vi "Autonomous Shooting.vi"(6 "Cross Obstacle":bool, 7 "Ball in place":bool, 8 "The Desired":T1={"Desired Angle"=45.0, "Desired Distance"=30.0, "Desired Time"=4.0}, 9 "Sensor Values":T2, 10 "Goal Selection":cluster{"High Goal":bool, "Low Goal":bool}, 11 "Position Selection":T6) -> (0 "Complete":bool, 1 "Arcada Drive?":bool, 2 "Tank Drive":T4, 3 "Aracade Drive":T5)   [LabVIEW 2015]
uses:
  Autonomous Shooting States.ctl
  Sensors.vi
panel:
  in  "Desired Angle for Position 2":dbl
  in  "Speed":dbl=0.4
  out "Set Roller/Shoot Motor":T3
  in  "X axis value":dbl=0.3
  # "12.27272727272727271"
  # "12.27272727272727271"
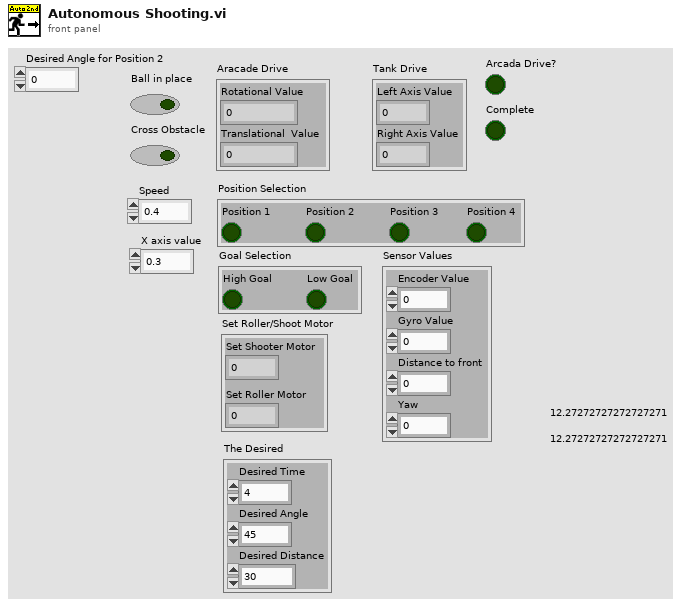
[diagram p1: front panel]
types:
  T1 = cluster{"Desired Angle":dbl, "Desired Distance":dbl, "Desired Time":dbl}
  T2 = cluster{"Encoder Value":dbl, "Gyro Value":dbl, "Distance to front":dbl, "Yaw":dbl}
  T3 = cluster{"Set Shooter Motor":dbl, "Set Roller Motor":dbl}
  T4 = cluster{"Left Axis Value":dbl, "Right Axis Value":dbl}
  T5 = cluster{"Rotational Value":dbl, "Translational  Value":dbl}
  T6 = cluster{"Position 1":bool, "Position 2":bool, "Position 3":bool, "Position 4":bool}
  T7 = typedef "Autonomous Shooting States.ctl" = enum16{"Ready", "Correct Heading", "Zero Encoder", "Drive Forward for X", "Turn towards goal 1", "Turn towards goal 2", "Turn towards goal 3", "Drive to Castle", "Check goal", "High Goal", "Positioning", "Low Goal", "Complete"}
  T8 = cluster{"Rotational Value":dbl, "Rotational Value":dbl}
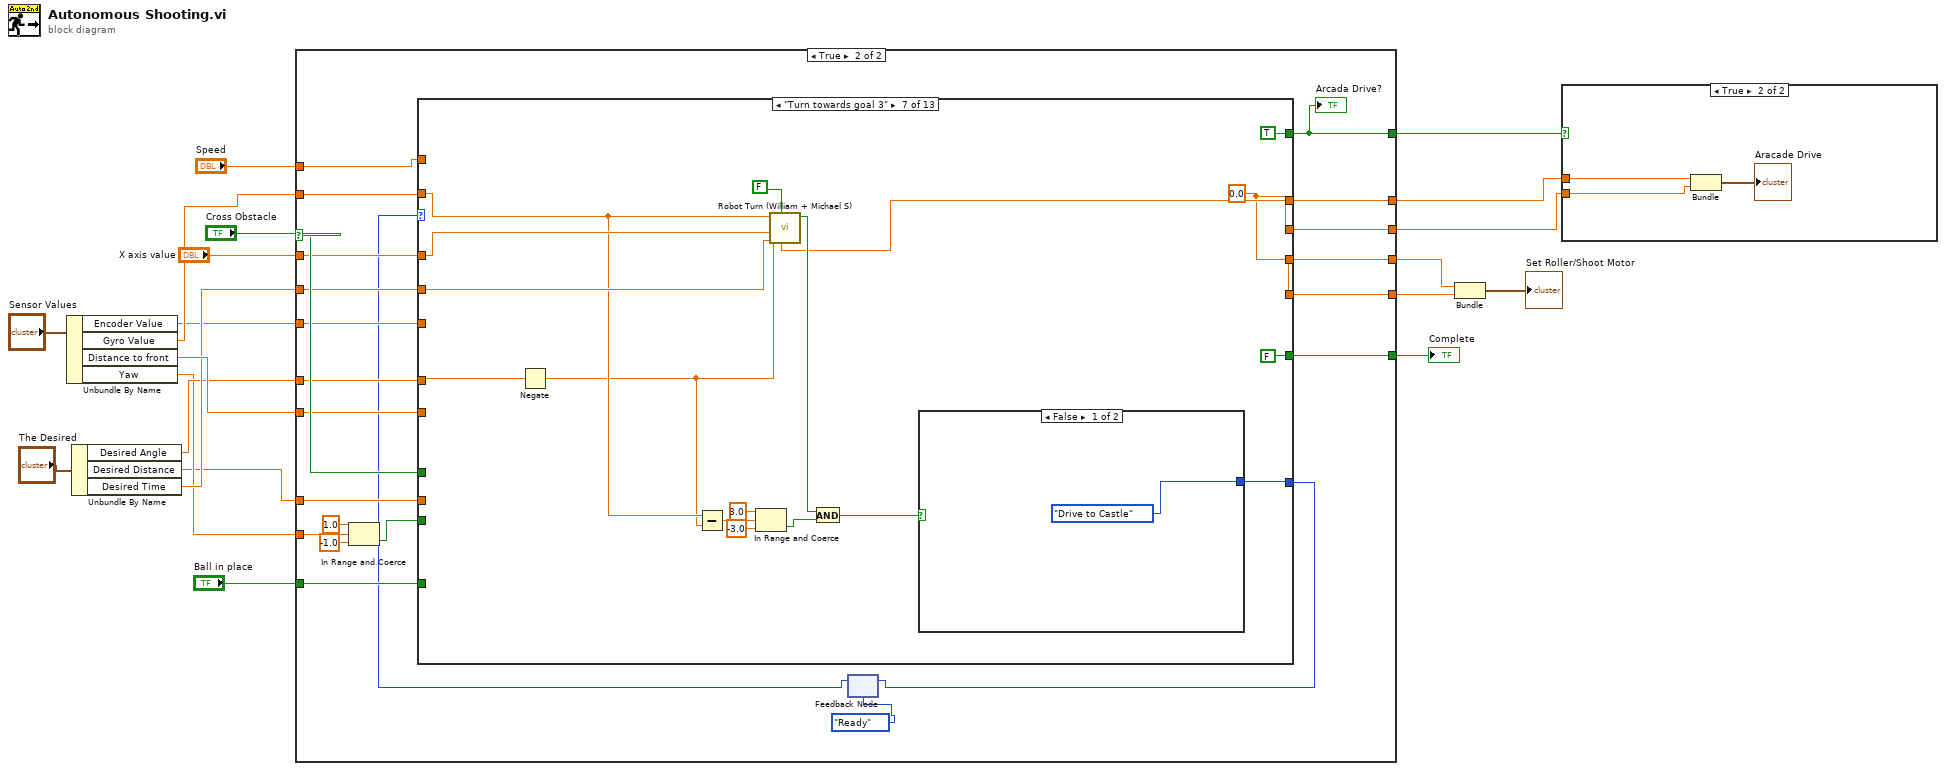
[diagram p0: block diagram]
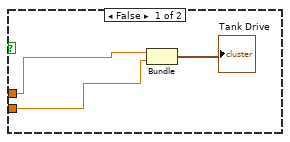
[diagram p2: hidden frame]
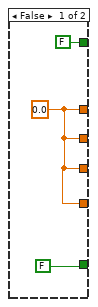
[diagram p3: hidden frame]
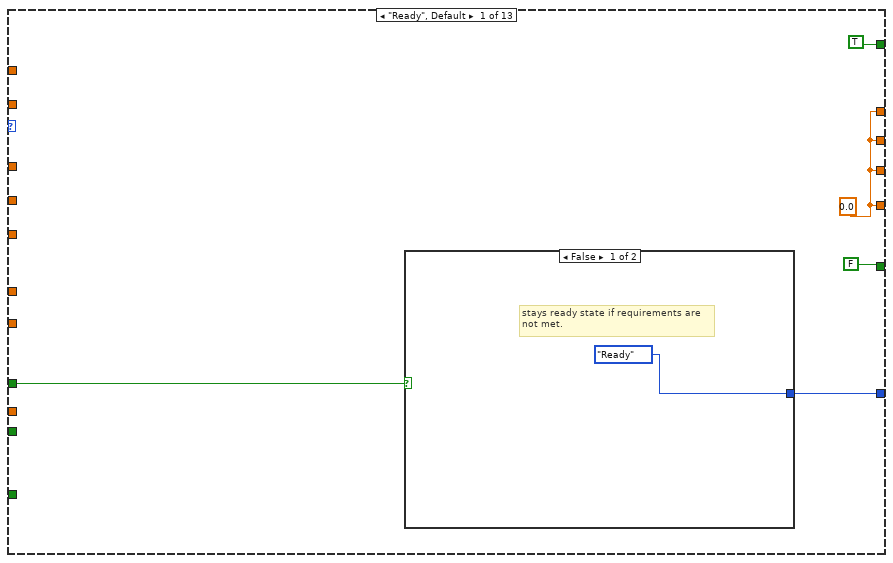
[diagram p4: hidden frame]
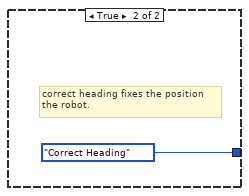
[diagram p5: hidden frame]
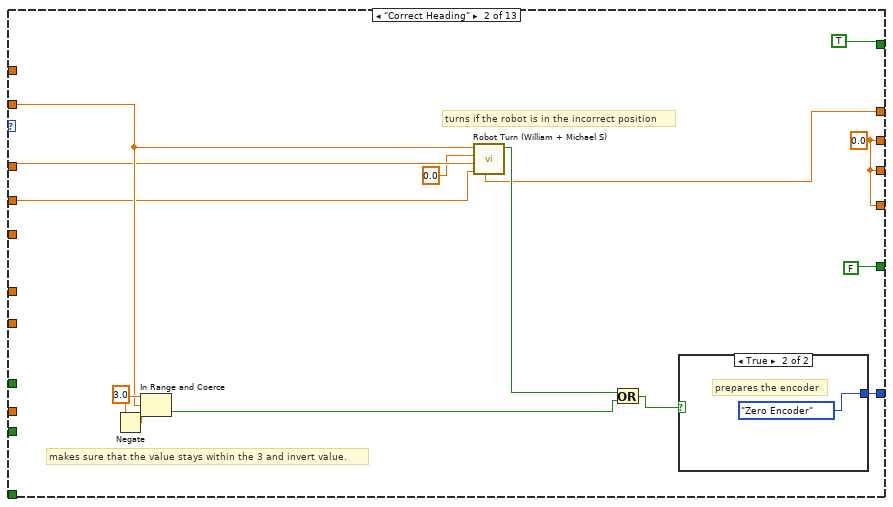
[diagram p6: hidden frame]
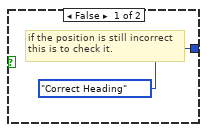
[diagram p7: hidden frame]
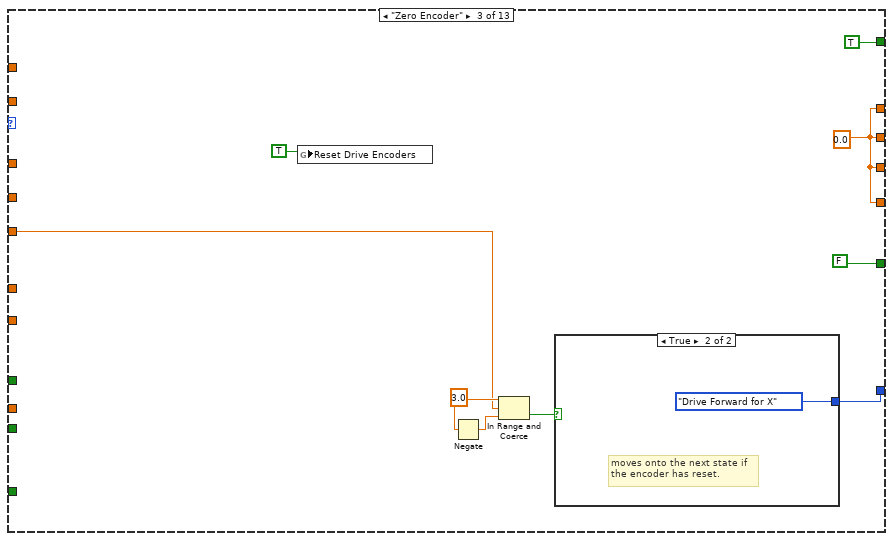
[diagram p8: hidden frame]
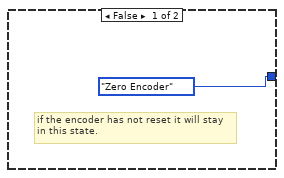
[diagram p9: hidden frame]
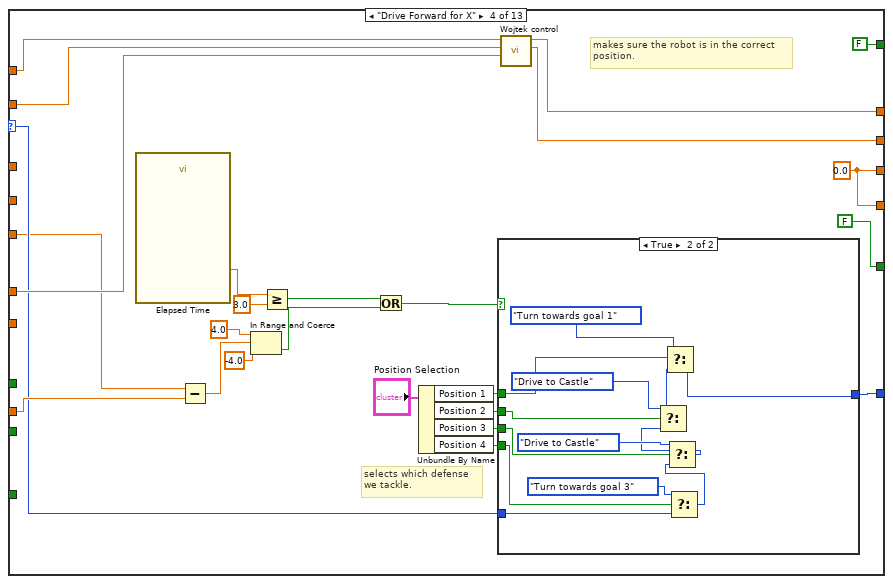
[diagram p10: hidden frame]
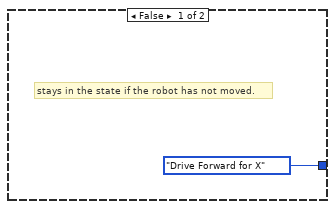
[diagram p11: hidden frame]
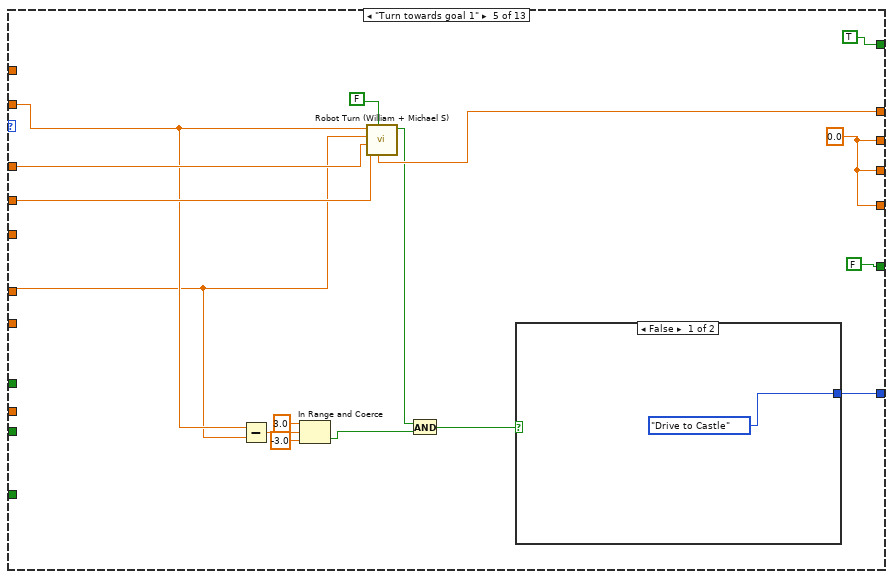
[diagram p12: hidden frame]
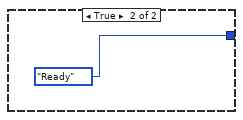
[diagram p13: hidden frame]
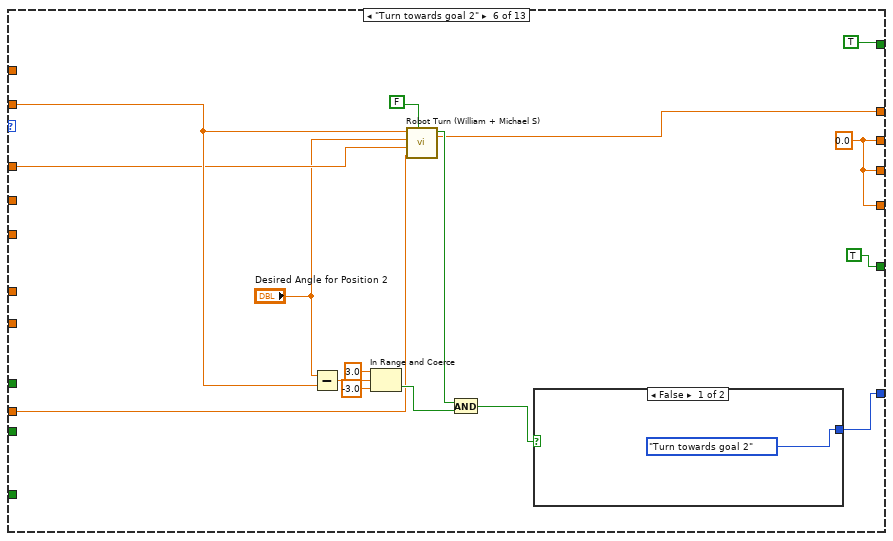
[diagram p14: hidden frame]
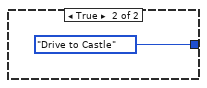
[diagram p15: hidden frame]
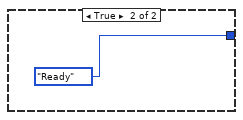
[diagram p16: hidden frame]
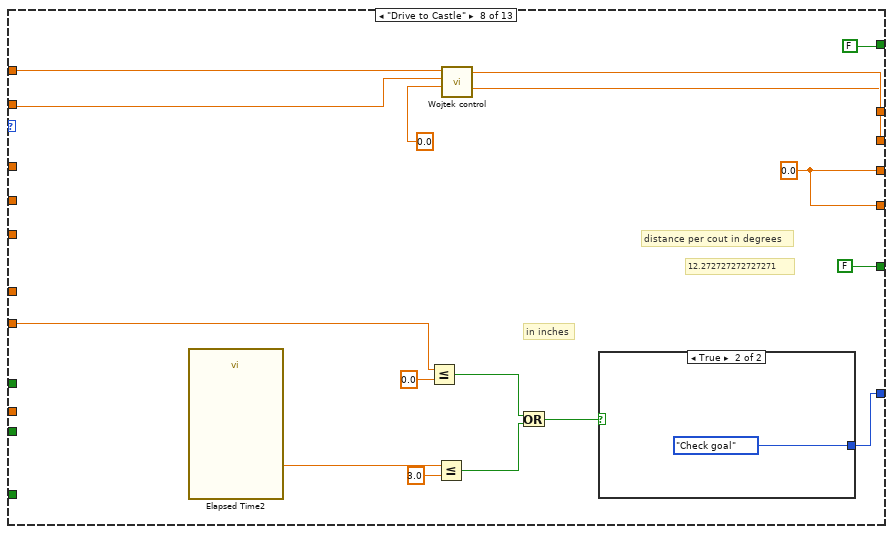
[diagram p17: hidden frame]
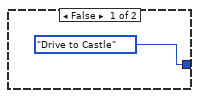
[diagram p18: hidden frame]
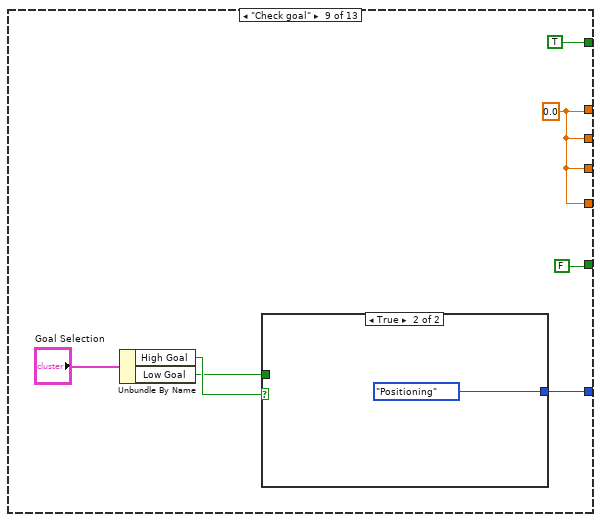
[diagram p19: hidden frame]
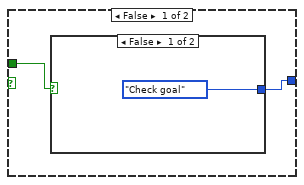
[diagram p20: hidden frame]
diagram:
  n1 = Unbundle By Name("Sensor Values") -> ("Encoder Value"=w1:dbl, "Gyro Value"=w9:dbl, "Distance to front"=w8:dbl, "Yaw"=w4:dbl)
  n2 = Unbundle By Name("The Desired") -> ("Desired Angle"=w5:dbl, "Desired Distance"=w3:dbl, "Desired Time"=w6:dbl)
  n3 = case shown="True" "Cross Obstacle" {
    selector: "Cross Obstacle" -> [_ w43]
    tunnel: [w22 w46] -> w15
    tunnel: [w22 w45] -> w14
    tunnel: [w22 w44] -> w13
    tunnel: w9 -> [_ w42]
    tunnel: w3 -> [_ w41]
    tunnel: w5 -> [_ w40]
    tunnel: w4 -> [_ w35]
    tunnel: "X axis value" -> [_ w39]
    tunnel: w6 -> [_ w38]
    tunnel: [w22 w33] -> w16
    tunnel: w8 -> [_ w32]
    tunnel: "Ball in place" -> [_ w31]
    tunnel: [FALSE w29] -> w17
    tunnel: "Speed" -> [_ w30]
    tunnel: [FALSE w28] -> w2
    tunnel: w1 -> [_ w27]
    frame False {
      w22 = 0.0
    }
    frame True {
      n4 = In Range and Coerce(upper limit=1.0, x=w35, lower limit=-1.0) -> (In Range?=w34:bool)  [unwired: 1 out]
      n5 = feedback #1(Autonomous_Shooting_States."Ready") -> (w25:T7)
      n6 = case shown="\"Turn towards goal 3\"" w25 {
        selector: w25 -> [_ _ _ w82 _ _ _ _ _ _ _ _ _]
        tunnel: [w49 w56 w74 w88 w127 w140 w165 w177 w195 w213 w224 0.5 w248] -> w46
        tunnel: [w49 w56 w74 w87 w127 w140 w165 w179 w195 0.9 0.75 w237 w248] -> w45
        tunnel: [w49 w56 w74 w87 w127 w140 w165 w179 w195 w205 0.0 1.0 w248] -> w44
        tunnel: [w51 w67 w75 w105 w135 w152 w164 w181 w197 w220 w231 w244 Autonomous_Shooting_States."Complete"] -> w24
        tunnel: w43 -> [w50 _ _ _ _ _ _ _ _ _ _ _ _]
        tunnel: w42 -> [_ w64 _ w85 w122 w145 w158 w190 _ _ _ _ _]
        tunnel: w41 -> [_ _ _ w101 _ w142 _ _ _ _ _ _ _]
        tunnel: w40 -> [_ _ _ w90 w121 _ w169 _ _ _ _ _ _]
        tunnel: [w49 w57 w74 w89 w134 w143 w168 w178 w195 w213 w224 w237 w248] -> w33
        tunnel: w39 -> [_ w63 _ _ w130 w144 w167 _ _ _ _ _ _]
        tunnel: w38 -> [_ w62 _ _ w129 _ w166 _ _ _ _ _ _]
        tunnel: w34 -> [_ _ _ _ _ _ _ _ _ _ _ _ _]
        tunnel: w32 -> [_ _ _ _ _ _ _ w188 _ _ _ _ _]
        tunnel: w31 -> [_ _ _ _ _ _ _ _ _ w216 _ w239 _]
        tunnel: [TRUE TRUE TRUE FALSE TRUE TRUE TRUE FALSE TRUE TRUE TRUE TRUE TRUE] -> w29
        tunnel: w30 -> [_ _ _ w84 _ _ _ w176 _ _ _ _ _]
        tunnel: [FALSE FALSE FALSE FALSE FALSE TRUE FALSE FALSE FALSE FALSE FALSE FALSE TRUE] -> w28
        tunnel: w27 -> [_ _ w70 w81 _ _ _ _ _ _ _ _ _]
        frame "Ready", Default {
          w49 = 0.0
          n7 = case shown="False" w50 {
            tunnel: [Autonomous_Shooting_States."Ready" Autonomous_Shooting_States."Correct Heading"] -> w51
            frame False {
              # "stays ready state if requirements are\nnot met."
            }
            frame True {
              # "correct heading fixes the position \nthe robot."
            }
          }
        }
        frame "Correct Heading" {
          w56 = 0.0 ("Translational Set Val")
          w66 = 3.0 ("upper limit")
          # "turns if the robot is in the incorrect position"
          # "makes sure that the value stays within the 3 and invert value."
          n8 = Negate(x=w66) -> (-x=w65:dbl)
          n9 = In Range and Coerce(upper limit=w66, x=w64, lower limit=w65) -> (In Range?=w58:bool)  [unwired: 1 out]
          n10 = call "Robot Turn (William + Michael S).vi"("Desired Time"=w62, "X axis value"=w63, "Desired Degree"=0.0, "Gyro Degrees"=w64) -> ("Stop"=w59:bool, "Rotational Value"=w57:dbl)  [unwired: 6 in]
          n11 = Or(x=w59, y=w58) -> (x .or. y?=w61:bool)
          n12 = case shown="True" w61 {
            tunnel: [Autonomous_Shooting_States."Correct Heading" Autonomous_Shooting_States."Zero Encoder"] -> w67
            frame False {
              # "if the position is still incorrect\nthis is to check it."
            }
            frame True {
              # "prepares the encoder"
            }
          }
        }
        frame "Zero Encoder" {
          w77 = 3.0 ("upper limit")
          w74 = 0.0
          n13 = global write "Sensors.vi" "Reset Drive Encoders"(TRUE) -> ()
          n14 = Negate(x=w77) -> (-x=w76:dbl)
          n15 = In Range and Coerce(upper limit=w77, x=w70, lower limit=w76) -> (In Range?=w78:bool)  [unwired: 1 out]
          n16 = case shown="True" w78 {
            tunnel: [Autonomous_Shooting_States."Zero Encoder" Autonomous_Shooting_States."Drive Forward for X"] -> w75
            frame False {
              # "if the encoder has not reset it will stay\nin this state."
            }
            frame True {
              # "moves onto the next state if\nthe encoder has reset."
            }
          }
        }
        frame "Drive Forward for X" {
          w87 = 0.0
          # "makes sure the robot is in the correct \nposition."
          # "selects which defense \nwe tackle."
          n17 = call "Elapsed Time"() -> ("Elapsed Time (s)"=w104:dbl)  [unwired: 12 in, 7 out]
          n18 = Subtract(x=w81, y=w101) -> (x-y=w100:dbl)
          n19 = In Range and Coerce(upper limit=4.0, x=w100, lower limit=-4.0) -> (In Range?=w97:bool)  [unwired: 1 out]
          n20 = Greater Or Equal?(x=w104, y=3.0) -> (x >= y?=w102:bool)
          n21 = Or(x=w102, y=w97) -> (x .or. y?=w91:bool)
          n22 = Unbundle By Name("Position Selection") -> ("Position 1"=w95:bool, "Position 2"=w94:bool, "Position 3"=w93:bool, "Position 4"=w92:bool)
          n23 = case shown="True" w91 {
            tunnel: [Autonomous_Shooting_States."Drive Forward for X" w114] -> w105
            tunnel: w95 -> [_ w119]
            tunnel: w94 -> [_ w117]
            tunnel: w93 -> [_ w112]
            tunnel: w92 -> [_ w110]
            tunnel: w82 -> [_ w108]
            frame False {
              # "stays in the state if the robot has not moved."
            }
            frame True {
              n24 = Select(t=Autonomous_Shooting_States."Turn towards goal 3", s=w110, f=w108) -> (s? t:f=w107:T7)
              n25 = Select(t=Autonomous_Shooting_States."Drive to Castle", s=w112, f=w107) -> (s? t:f=w111:T7)
              n26 = Select(t=Autonomous_Shooting_States."Drive to Castle", s=w117, f=w111) -> (s? t:f=w115:T7)
              n27 = Select(t=Autonomous_Shooting_States."Turn towards goal 1", s=w119, f=w115) -> (s? t:f=w114:T7)
            }
          }
          n28 = call "Wojtek control.vi"("Desired Angle"=w90, "Gyro Angle"=w85, "Speed"=w84) -> ("right axis value"=w88:dbl, "left axis value"=w89:dbl)  [unwired: 7 in]
        }
        frame "Turn towards goal 1" {
          w127 = 0.0
          n29 = Subtract(x=w122, y=w121) -> (x-y=w125:dbl)
          n30 = In Range and Coerce(upper limit=3.0, x=w125, lower limit=-3.0) -> (In Range?=w120:bool)  [unwired: 1 out]
          n31 = call "Robot Turn (William + Michael S).vi"("Reset"=FALSE, "Desired Time"=w129, "X axis value"=w130, "Desired Degree"=w121, "Gyro Degrees"=w122) -> ("Stop"=w132:bool, "Rotational Value"=w134:dbl)  [unwired: 5 in]
          n32 = And(x=w132, y=w120) -> (x .and. y?=w131:bool)
          n33 = case shown="False" w131 {
            tunnel: [Autonomous_Shooting_States."Drive to Castle" Autonomous_Shooting_States."Ready"] -> w135
            frame False {
            }
            frame True {
            }
          }
        }
        frame "Turn towards goal 2" {
          w140 = 0.0 ("Rotational Value")
          n34 = Subtract(x="Desired Angle for Position 2", y=w145) -> (x-y=w151:dbl)
          n35 = In Range and Coerce(upper limit=3.0, x=w151, lower limit=-3.0) -> (In Range?=w148:bool)  [unwired: 1 out]
          n36 = call "Robot Turn (William + Michael S).vi"("Reset"=FALSE, "Desired Time"=w142, "X axis value"=w144, "Desired Degree"="Desired Angle for Position 2", "Gyro Degrees"=w145) -> ("Stop"=w147:bool, "Rotational Value"=w143:dbl)  [unwired: 5 in]
          n37 = And(x=w147, y=w148) -> (x .and. y?=w146:bool)
          n38 = case shown="False" w146 {
            tunnel: [Autonomous_Shooting_States."Turn towards goal 2" Autonomous_Shooting_States."Drive to Castle"] -> w152
            frame False {
            }
            frame True {
            }
          }
        }
        frame "Turn towards goal 3" {
          w165 = 0.0
          n39 = Negate(x=w169) -> (-x=w157:dbl)
          n40 = Subtract(x=w158, y=w157) -> (x-y=w161:dbl)
          n41 = In Range and Coerce(upper limit=3.0, x=w161, lower limit=-3.0) -> (In Range?=w156:bool)  [unwired: 1 out]
          n42 = call "Robot Turn (William + Michael S).vi"("Reset"=FALSE, "Desired Time"=w166, "X axis value"=w167, "Desired Degree"=w157, "Gyro Degrees"=w158) -> ("Stop"=w171:bool, "Rotational Value"=w168:dbl)  [unwired: 5 in]
          n43 = And(x=w171, y=w156) -> (x .and. y?=w170:bool)
          n44 = case shown="False" w170 {
            tunnel: [Autonomous_Shooting_States."Drive to Castle" Autonomous_Shooting_States."Ready"] -> w164
            frame False {
            }
            frame True {
            }
          }
        }
        frame "Drive to Castle" {
          w179 = 0.0
          # "distance per cout in degrees"
          # "in inches"
          # "12.272727272727271"
          n45 = call "Elapsed Time2"() -> ("Elapsed Time (s)"=w186:dbl)  [unwired: 12 in, 7 out]
          n46 = Less Or Equal?(x=w188, y=0.0) -> (x <= y?=w184:bool)
          n47 = Less Or Equal?(x=w186, y=3.0) -> (x <= y?=w183:bool)
          n48 = call "Wojtek control.vi"("Desired Angle"=0.0, "Gyro Angle"=w190, "Speed"=w176) -> ("right axis value"=w177:dbl, "left axis value"=w178:dbl)  [unwired: 7 in]
          n49 = Or(x=w184, y=w183) -> (x .or. y?=w182:bool)
          n50 = case shown="True" w182 {
            tunnel: [Autonomous_Shooting_States."Drive to Castle" Autonomous_Shooting_States."Check goal"] -> w181
            frame False {
            }
            frame True {
            }
          }
        }
        frame "Check goal" {
          w195 = 0.0
          n51 = Unbundle By Name("Goal Selection") -> ("High Goal"=w198:bool, "Low Goal"=w196:bool)
          n52 = case shown="True" w198 {
            tunnel: [w200 Autonomous_Shooting_States."Positioning"] -> w197
            tunnel: w196 -> [w201 _]
            frame False {
              n53 = case shown="False" w201 {
                tunnel: [Autonomous_Shooting_States."Check goal" Autonomous_Shooting_States."Low Goal"] -> w200
                frame False {
                }
                frame True {
                }
              }
            }
            frame True {
            }
          }
        }
        frame "High Goal" {
          w213 = 0.0
          n54 = call "Elapsed Time5"() -> ("Elapsed Time (s)"=w219:dbl)  [unwired: 12 in, 7 out]
          n55 = Greater Or Equal?(x=w219, y=2.5) -> (x >= y?=w217:bool)
          n56 = global read "Sensors.vi" "Shooter Speed"() -> (w210:dbl)
          n57 = Greater Or Equal?(x=w210, y=22000.0) -> (x >= y?=w208:bool)
          n58 = And(x=w217, y=w216) -> (x .and. y?=w215:bool)
          n59 = Select(t=-1.0, s=w208, f=0.0) -> (s? t:f=w205:dbl)
          n60 = case shown="True" w215 {
            tunnel: [Autonomous_Shooting_States."High Goal" Autonomous_Shooting_States."Complete"] -> w220
            frame False {
            }
            frame True {
            }
          }
        }
        frame "Positioning" {
          w224 = 0.0 ("Rotational Value")
          n61 = call "Elapsed Time3"() -> ("Elapsed Time (s)"=w230:dbl)  [unwired: 12 in, 7 out]
          n62 = Greater Or Equal?(x=w230, y=4.0) -> (x >= y?=w223:bool)
          n63 = case shown="True" w223 {
            tunnel: [Autonomous_Shooting_States."Positioning" Autonomous_Shooting_States."High Goal"] -> w231
            frame False {
            }
            frame True {
            }
          }
        }
        frame "Low Goal" {
          w237 = 0.0
          n64 = call "Elapsed Time4"() -> ("Elapsed Time (s)"=w243:dbl)  [unwired: 12 in, 7 out]
          n65 = Greater?(x=w243, y=3.0) -> (0:w240:bool)
          n66 = And(x=w240, y=w239) -> (x .and. y?=w238:bool)
          n67 = case shown="False" w238 {
            tunnel: [Autonomous_Shooting_States."Low Goal" Autonomous_Shooting_States."Complete"] -> w244
            frame False {
            }
            frame True {
            }
          }
        }
        frame "Complete" {
          w248 = 0.0
        }
      }
      "Arcada Drive?" <- w29
      n68 = feedback-in #1(w24) -> ()
    }
  }
  "Complete" <- w2
  n69 = Bundle("Rotational Value"=w14, "f"=w13) -> (→"Set Roller/Shoot Motor":cluster{"Rotational Value":dbl, "f":dbl})  [unwired: 1 in]
  n70 = case shown="True" w17 {
    tunnel: w16 -> [w253 w255]
    tunnel: w15 -> [w252 w256]
    frame False {
      n71 = Bundle("Rotational Value"=w253, "Rotational Value"=w252) -> (→"Tank Drive":T8)  [unwired: 1 in]
    }
    frame True {
      n72 = Bundle("Rotational Value"=w255, "Rotational Value"=w256) -> (→"Aracade Drive":T8)  [unwired: 1 in]
    }
  }
